vi "Status.vi"(8 "error in (no error)":errorcluster, 11 "Notifier in":refnum<class "Notifier.lvclass">) -> (0 "error out":errorcluster, 2 "Data Notification":refnum<class "Data.lvclass">, 3 "Notifier out":refnum<class "Notifier.lvclass">)   [LabVIEW 2020, in "Data.lvlib" / "Notifier.lvclass"]
doc: "Get the notifier status."
uses:
  Notifier.lvclass
  Data.lvclass
  Notifier.lvclass/Notifier.ctl
panel:
  out "# waiting":i32
  out "Notifier name":string
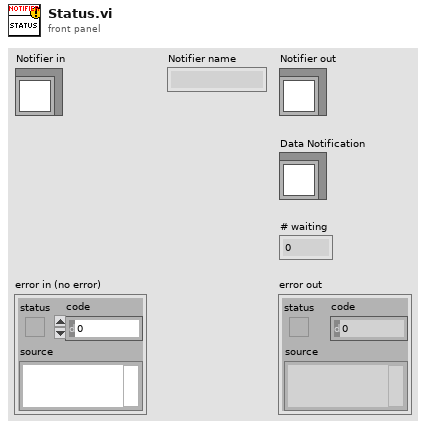
[diagram p1: front panel]
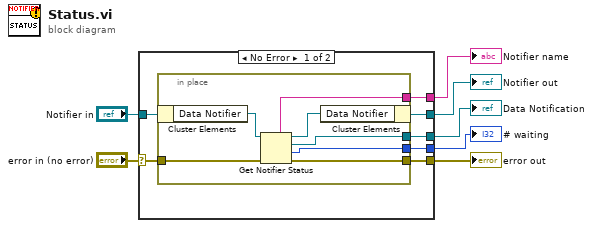
[diagram p0: block diagram]
diagram:
  n1 = case shown="No Error" "error in (no error)" {
    selector: "error in (no error)" -> [w12 w23]
    tunnel: [w11 w23] -> w6
    tunnel: [w13 w22] -> w4
    tunnel: "Notifier in" -> [w14 w22]
    tunnel: [w10 _] -> w3
    tunnel: [w9 _] -> w2
    tunnel: [w8 _] -> w1
    frame No Error {
      n2 = in-place {
        in-place-border: w12 -> [w17]
        in-place-border: [w19] -> w11
        in-place-border: [w18] -> w10
        in-place-border: [w16] -> w9
        in-place-border: [w15] -> w8
        n3 = in-place-cluster #1(w14) -> ("Data Notifier"=w21:refnum<notifier>)
        n4 = Get Notifier Status(notifier=w21, error in (no error)=w17) -> (notifier out=w20:refnum<notifier>, notifier name=w16:string, current notification=w18:refnum<class "Data.lvclass">, # waiting=w15:i32, error out=w19:errorcluster)
        n5 = in-place-cluster #1("Data Notifier"=w20) -> (w13:refnum<class "Notifier.lvclass">)
      }
    }
    frame Error {
    }
  }
  "error out" <- w6
  "Notifier out" <- w4
  "Data Notification" <- w3
  "# waiting" <- w1
  "Notifier name" <- w2
